vi "Initialize.vi"(6 "optional":variant, 8 "error in":errorcluster, 11 "Packet in":refnum<class "Packet.lvclass">) -> (0 "error out":errorcluster, 3 "Node*":refnum<data-value>)   [LabVIEW 2013, in "Packet.lvclass"]
doc: "Initializes a node. Makes a data value reference of the node, sets the selfNode, and output the data value reference."
uses:
  Packet.lvclass
  xCE/xceNode/xceNode.lvclass
  xCE/xceDataNode/xceDataNode.lvclass
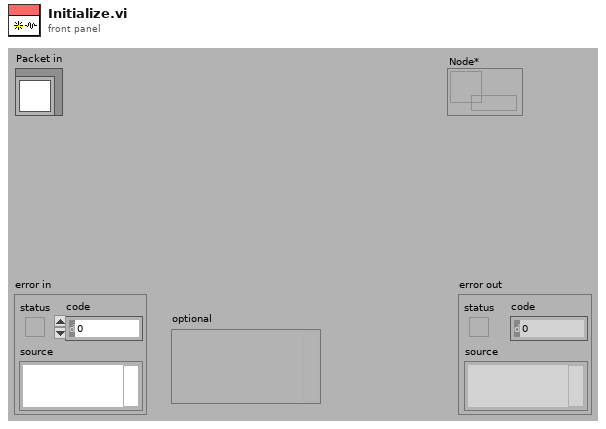
[diagram p1: front panel]
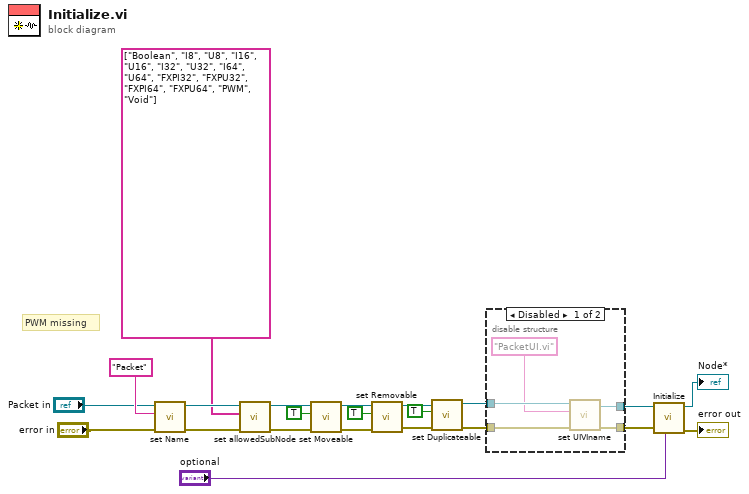
[diagram p0: block diagram]
diagram:
  # "PWM missing"
  n1 = call "set Name.vi"("error in (no error)"="error in", "Name"="Packet", "xceDataNode in"="Packet in") -> ("error out"=w18:errorcluster, "xceDataNode out"=w19:refnum<class "Packet.lvclass">)  [unwired: 7 in]
  n2 = call "set allowedSubNode.vi"("error in (no error)"=w18, "Allowed subNode[]"=string[] ["Boolean", "I8", "U8", "I16", "U16", "I32", "U32", "I64", "U64", "FXPI32", "FXPU32", "FXPI64", "FXPU64", "PWM", "Void"], "xceDataNode in"=w19) -> ("error out"=w13:errorcluster, "xceDataNode out"=w14:refnum<class "Packet.lvclass">)  [unwired: 7 in]
  n3 = call "set Moveable.vi"("error in (no error)"=w13, "Moveable"=TRUE, "xceDataNode in"=w14) -> ("error out"=w10:errorcluster, "xceDataNode out"=w11:refnum<class "Packet.lvclass">)  [unwired: 7 in]
  n4 = call "set Removable.vi"("error in (no error)"=w10, "Removable"=TRUE, "xceDataNode in"=w11) -> ("error out"=w7:errorcluster, "xceDataNode out"=w8:refnum<class "Packet.lvclass">)  [unwired: 7 in]
  n5 = call "set Duplicateable.vi"("error in (no error)"=w7, "Duplicateable"=TRUE, "xceDataNode in"=w8) -> ("error out"=w4:errorcluster, "xceDataNode out"=w5:refnum<class "Packet.lvclass">)  [unwired: 7 in]
  n6 = disable-structure shown="Disabled" {
    disable-tunnel: w5 -> [w27 w29]
    disable-tunnel: w4 -> [w26 w28]
    disable-tunnel: [w25 w29] -> w3
    disable-tunnel: [w24 w28] -> w2
    frame Disabled {
      n7 = call "set UIVIname.vi"("error in (no error)"=w26, "UI VI name"="PacketUI.vi", "xceDataNode in"=w27) -> ("error out"=w24:errorcluster, "xceDataNode out"=w25:refnum<class "Packet.lvclass">)  [unwired: 7 in]
    }
    frame Enabled {
    }
  }
  n8 = call-parent "Initialize.vi"("optional"="optional", "error in"=w2, "xceDataNode in"=w3) -> ("error out"=→"error out":errorcluster, "Node*"=→"Node*":refnum<data-value>)  [unwired: 7 in]
